vi "Analyze.vi"(8 "error in (no error)":errorcluster, 11 "HIJ Vision Display in":refnum<class "HIJ Vision Display.lvclass">) -> (0 "error out":errorcluster, 3 "HIJ Vision Display out":refnum<class "HIJ Vision Display.lvclass">)   [LabVIEW 2020, in "HIJ Vision Display.lvlib" / "HIJ Vision Display.lvclass"]
uses:
  HIJ Vision Display.lvclass
  <vilib>/vision/Image Controls.llb/IMAQ Image.ctl
  HIJ Vision Display.lvclass/HIJ Vision Display.ctl
  Analyze/Analyze Actor/Analyze Actor Messages/Analyze Msg/Analyze Msg.lvclass/Analyze Msg.ctl
  <vilib>/ActorFramework/Message Enqueuer/Message Enqueuer.lvclass/Message Enqueuer.ctl
  <vilib>/ActorFramework/Message Enqueuer/Enqueue.vi
  Analyze/Analyze Actor/Analyze Actor Messages/Analyze Msg/Analyze Msg.lvclass
  C:/Program Files (x86)/National Instruments/LabVIEW 2020/vi.lib/ActorFramework/Message/Message.lvclass
  <vilib>/ActorFramework/Message Priority Queue/Priority Enqueue.vi
  <vilib>/ActorFramework/Message Enqueuer/Message Enqueuer.lvclass
panel:
  out "Image Out":T1
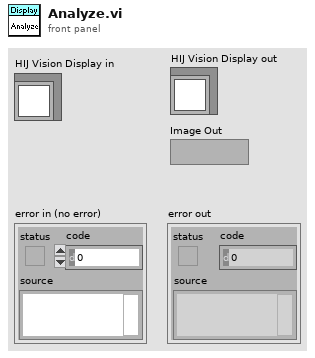
[diagram p1: front panel]
types:
  T1 = typedef "IMAQ Image.ctl" = refnum<image>
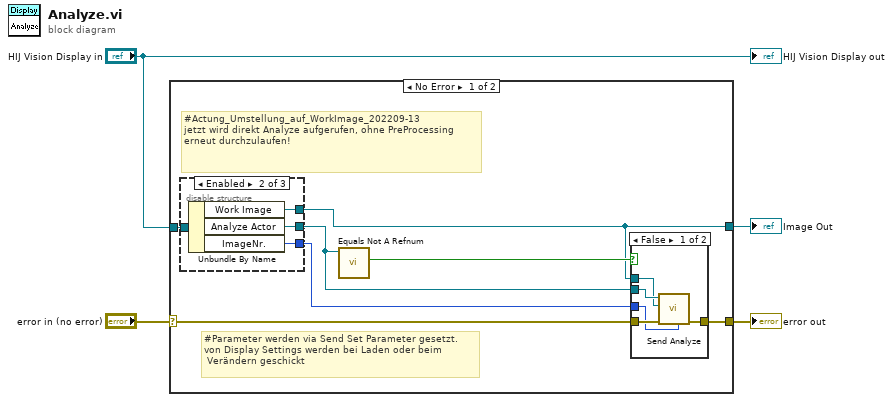
[diagram p0: block diagram]
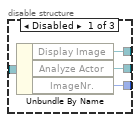
[diagram p2: hidden frame]
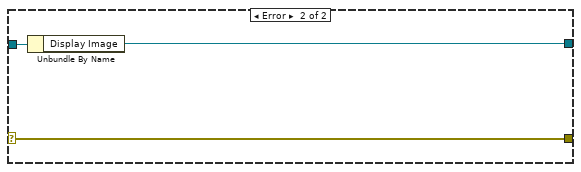
[diagram p5: hidden frame]
diagram:
  n1 = case shown="No Error" "error in (no error)" {
    selector: "error in (no error)" -> [w7 w28]
    tunnel: [w11 w28] -> w4
    tunnel: "HIJ Vision Display in" -> [w8 w27]
    tunnel: [w5 w26] -> w1
    frame No Error {
      # "#Actung_Umstellung_auf_WorkImage_202209-13\njetzt wird direkt Analyze aufgerufen, ohne PreProcessing\nerneut durchzulaufen!"
      # "#Parameter werden via Send Set Parameter gesetzt.\nvon Display Settings werden bei Laden oder beim\n Verändern geschickt"
      n2 = disable-structure shown="Enabled" {
        disable-tunnel: [w15 w19 _] -> w10
        disable-tunnel: [w14 w18 _] -> w9
        disable-tunnel: w8 -> [w13 w17 _]
        disable-tunnel: [w12 w16 _] -> w5
        frame Disabled {
          n3 = Unbundle By Name(w13) -> ("Display Image"=w12:T1, "Analyze Actor"=w15:refnum<class "Message Enqueuer.lvclass">, "ImageNr."=w14:i32)
        }
        frame Enabled {
          n4 = Unbundle By Name(w17) -> ("Work Image"=w16:T1, "Analyze Actor"=w19:refnum<class "Message Enqueuer.lvclass">, "ImageNr."=w18:i32)
        }
        frame Disabled {
        }
      }
      n5 = call <vilib>:"Equals Not A Refnum.vi"("Message Enqueuer"=w10) -> ("Not a refnum?"=w6:bool)  [unwired: 10 in]
      n6 = case shown="False" w6 {
        tunnel: w10 -> [w24 _]
        tunnel: w5 -> [w23 _]
        tunnel: w7 -> [w22 w25]
        tunnel: [w21 w25] -> w11
        tunnel: w9 -> [w20 _]
        frame False {
          n7 = call "Send Analyze.vi"("Image Nr."=w20, "error in (no error)"=w22, "Image"=w23, "Message Enqueuer"=w24) -> ("error out"=w21:errorcluster)  [unwired: 6 in, 1 out]
        }
        frame True {
        }
      }
    }
    frame Error {
      n8 = Unbundle By Name(w27) -> ("Display Image"=w26:T1)
    }
  }
  "error out" <- w4
  "Image Out" <- w1
  "HIJ Vision Display out" <- "HIJ Vision Display in"
